vi "Send Synchronous Message.vi"(6 "Wait timeout in ms (-1)":i32=-1, 8 "error in (no error)":errorcluster, 9 "Message Priority (Normal)":T1=enum."Normal", 10 "SynchronousMsg In":refnum<class "SynchronousMsg.lvclass">, 11 "Message Enqueuer In":refnum<class "Message Enqueuer.lvclass">) -> (0 "error out":errorcluster, 1 "Actor Return Error":errorcluster, 2 "Data":variant, 3 "Message Enqueuer Out":refnum<class "Message Enqueuer.lvclass">)   [LabVIEW 2015, in "AbstractMessages.lvlib" / "SynchronousMsg.lvclass"]
doc: "<License>\nCopyright © 2017 Composed Systems, LLC | All rights reserved\nwww.composed.io\n\nAuthor: Ethan Stern <ethan.stern@composed.io>\n\nThis software is provided \"AS IS\" WITHOUT WARRANTIES, either express or implied, AND IS FOR EDUCATIONAL PURPOSES ONLY.\n</License>"
uses:
  SynchronousMsg.lvclass
  <vilib>/ActorFramework/Message Enqueuer/Message Enqueuer.lvclass
  <vilib>/ActorFramework/Message Enqueuer/Message Priority.ctl
  SynchronousMsg.lvclass/SynchronousMsg.ctl
  <vilib>/ActorFramework/Message Enqueuer/Message Enqueuer.lvclass/Message Enqueuer.ctl
  <vilib>/ActorFramework/Message Priority Queue/Priority Enqueue.vi
  <vilib>/ErrorRing/Error Ring.xnode
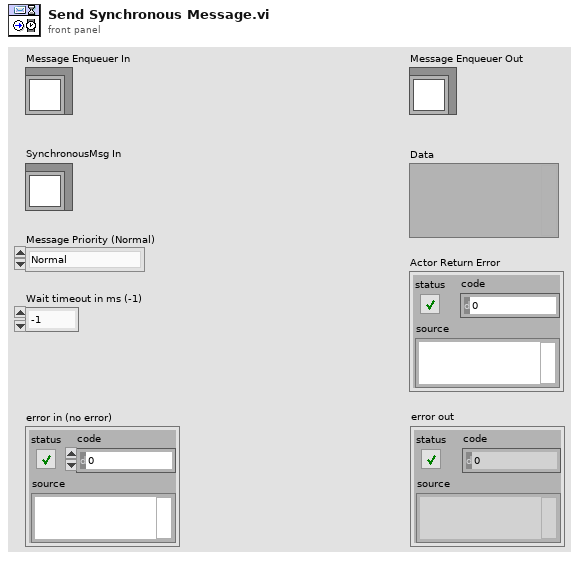
[diagram p1: front panel]
types:
  T1 = typedef "Actor Framework.lvlib/Message Enqueuer.lvclass/Message Priority.ctl" = enum16{"Low", "Normal", "High"}
  T2 = cluster{"Data":variant, "Return Error":errorcluster}
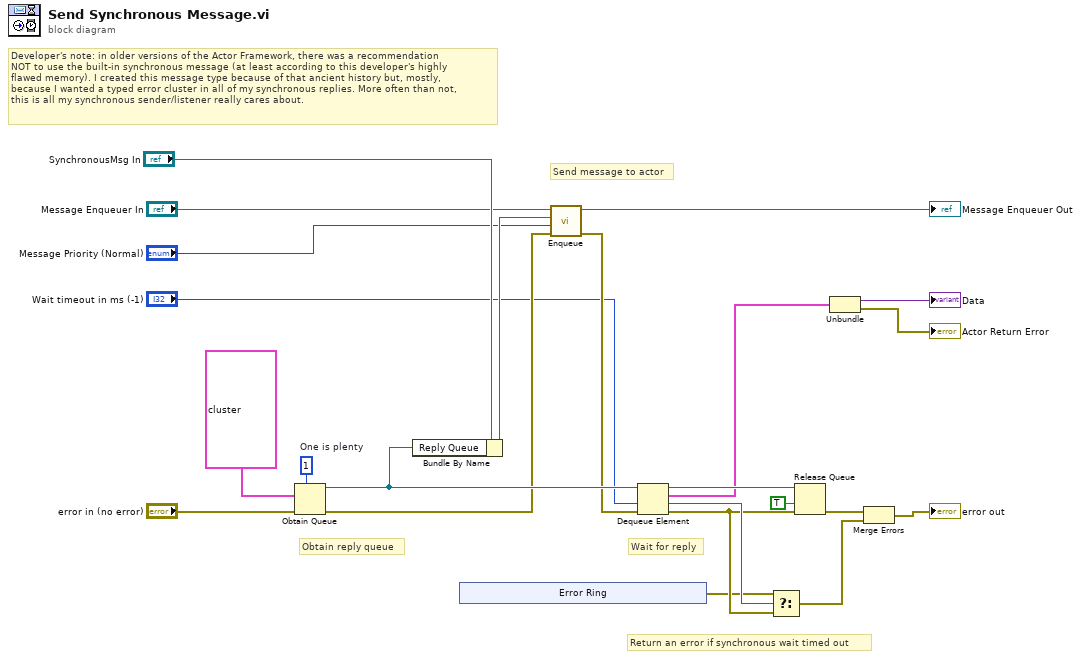
[diagram p0: block diagram]
diagram:
  w20 = 1  # One is plenty
  # "Return an error if synchronous wait timed out"
  # "Obtain reply queue"
  # "Wait for reply"
  # "Send message to actor"
  # "Developer's note: in older versions of the Actor Framework, there was a recommendation\nNOT to use the built-in synchronous message (at least according to this developer's highly\nflawed memory). I created this message type because of that ancient history but, mostly, \nbecause I wanted a typed error cluster in all of my synchronous replies. More often than not,\nthis is all my synchronous sender/listener really cares about."
  n1 = Obtain Queue(max queue size (-1, unlimited)=w20, element data type=T2 {"Data"=variant, "Return Error"={"status"=FALSE, "code"=0, "source"=""}}, error in (no error)="error in (no error)") -> (queue out=w23:refnum<queue>, error out=w18:errorcluster)  [unwired: 2 in, 1 out]
  n2 = Bundle By Name(cluster="SynchronousMsg In", "Reply Queue"=w23) -> (w17:refnum<class "SynchronousMsg.lvclass">)
  n3 = xnode "Error Ring"() -> ("error out"=w3:errorcluster)
  n4 = call <vilib>:"Enqueue.vi"("error in (no error)"=w18, "Message Priority (Normal)"="Message Priority (Normal)", "Message"=w17, "Message Enqueuer in"="Message Enqueuer In") -> ("error out"=w15:errorcluster, "Message Enqueuer out"=→"Message Enqueuer Out":refnum<class "Message Enqueuer.lvclass">)  [unwired: 6 in]
  n5 = Dequeue Element(queue=w23, timeout in ms (-1)="Wait timeout in ms (-1)", error in (no error)=w15) -> (queue out=w14:refnum<queue>, element=w10:T2, timed out?=w5:bool, error out=w4:errorcluster)
  n6 = Select(t=w3, s=w5, f=w4) -> (s? t:f=w1:errorcluster)
  n7 = Release Queue(queue=w14, force destroy? (F)=TRUE, error in (no error)=w4) -> (error out=w13:errorcluster)  [unwired: 2 out]
  n8 = Unbundle(w10) -> ("Data"=→"Data":variant, "Return Error"=→"Actor Return Error":errorcluster)
  n9 = Merge Errors(w13, w1) -> (→"error out":errorcluster)
